vi "Main.RTM.AddWaveforms.vi"(8 "error in (no error)":errorcluster, 11 "Node Ptr":u64 format="%.0x") -> (0 "error out":errorcluster)   [LabVIEW 2015, in "Waveform-Processing-Custom-Device System Explorer.lvlib"]
uses:
  Waveform-Processing-Custom-Device System Explorer.lvlib
  NationalInstruments.VeriStand.SystemStorageUI
  <vilib>/NI Veristand/UI Controls/System Definition Tree/NI_VS UI System Tree.lvlib
panel:
  in  "TreeBrowserWF":refnum<k24>(container)
  in  "Tag":string
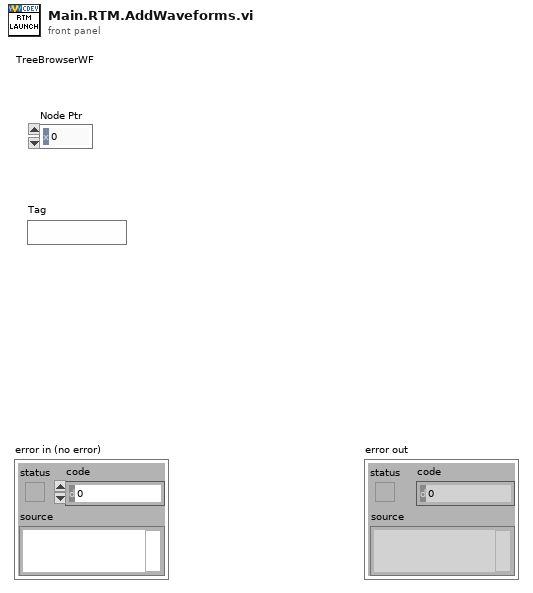
[diagram p1: front panel]
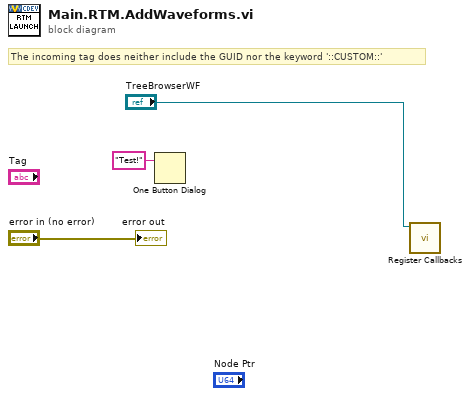
[diagram p0: block diagram]
diagram:
  # "The incoming tag does neither include the GUID nor the keyword '::CUSTOM::'"
  n1 = One Button Dialog(message="Test!") -> ()  [unwired: 1 in, 1 out]
  n2 = call <vilib>:"Register Callbacks.vi"("System Definition Tree"="TreeBrowserWF") -> ()  [unwired: 8 in, 3 out]
  "error out" <- "error in (no error)"
